vi "CRYCompare X-axis range.vi"(11 "Curves in":cluster{"x":dbl, "y":dbl, "z":dbl}[][](array[cluster])) -> (3 "All equal?":bool)   [LabVIEW 2013]
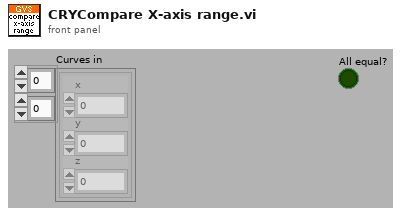
[diagram p1: front panel]
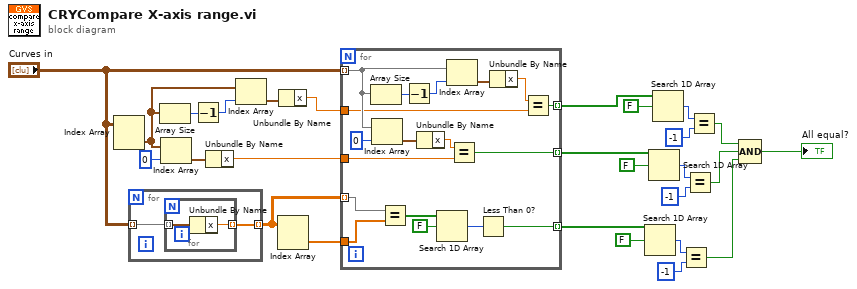
[diagram p0: block diagram]
diagram:
  n1 = Index Array(array="Curves in") -> (element=w23:cluster{"x":dbl, "y":dbl, "z":dbl}[])  [unwired: 2 in]
  n2 = for {
    tunnel: "Curves in" -> [w29] mode=indexing
    tunnel: [w28] -> w6 mode=indexing
    n3 = for {
      tunnel: w29 -> [w31] mode=indexing
      tunnel: [w30] -> w28 mode=indexing
      n4 = Unbundle By Name(w31) -> ("x"=w30:dbl)
    }
  }
  n5 = Array Size(array=w23) -> (size(s)=w25:i32)
  n6 = Index Array(array=w23, index=0) -> (element=w26:cluster{"x":dbl, "y":dbl, "z":dbl})
  n7 = Decrement(x=w25) -> (x-1=w24:i32)
  n8 = Unbundle By Name(w26) -> ("x"=w20:dbl)
  n9 = Index Array(array=w23, index=w24) -> (element=w22:cluster{"x":dbl, "y":dbl, "z":dbl})
  n10 = Index Array(array=w6) -> (element=w7:dbl[])  [unwired: 2 in]
  n11 = Unbundle By Name(w22) -> ("x"=w21:dbl)
  n12 = for {
    tunnel: "Curves in" -> [w44] mode=indexing
    tunnel: w21 -> [w40]
    tunnel: w20 -> [w42]
    tunnel: [w39] -> w12 mode=indexing
    tunnel: [w38] -> w13 mode=indexing
    tunnel: w7 -> [w36]
    tunnel: w6 -> [w37] mode=indexing
    tunnel: [w32] -> w2 mode=indexing
    n13 = Array Size(array=w44) -> (size(s)=w47:i32)
    n14 = Index Array(array=w44, index=0) -> (element=w46:cluster{"x":dbl, "y":dbl, "z":dbl})
    n15 = Equal?(x=w37, y=w36) -> (x = y?=w35:bool[])
    n16 = Decrement(x=w47) -> (x-1=w48:i32)
    n17 = Unbundle By Name(w46) -> ("x"=w43:dbl)
    n18 = Search 1D Array(1D array=w35, element=FALSE) -> (index of element=w33:i32)  [unwired: 1 in]
    n19 = Index Array(array=w44, index=w48) -> (element=w49:cluster{"x":dbl, "y":dbl, "z":dbl})
    n20 = Equal?(x=w43, y=w42) -> (x = y?=w38:bool)
    n21 = Less Than 0?(x=w33) -> (x < 0?=w32:bool)
    n22 = Unbundle By Name(w49) -> ("x"=w41:dbl)
    n23 = Equal?(x=w41, y=w40) -> (x = y?=w39:bool)
  }
  n24 = Search 1D Array(1D array=w2, element=FALSE) -> (index of element=w5:i32)  [unwired: 1 out]
  n25 = Search 1D Array(1D array=w13, element=FALSE) -> (index of element=w14:i32)  [unwired: 1 out]
  n26 = Search 1D Array(1D array=w12, element=FALSE) -> (index of element=w19:i32)  [unwired: 1 out]
  n27 = Equal?(x=w5, y=-1) -> (x = y?=w1:bool)
  n28 = Equal?(x=w14, y=-1) -> (x = y?=w10:bool)
  n29 = Equal?(x=w19, y=-1) -> (x = y?=w11:bool)
  n30 = Compound Arithmetic op=AND(w11, w10, w1) -> (→"All equal?":bool)
